vi "clusterUnderstanding.vi"() -> ()   [LabVIEW 2019]
panel:
  out "Numeric":dbl
  in  "Person  turn":dbl
  out "LED Two":bool
  out "Name":string
  out "Age":dbl
  out "LED One":bool
  in  "Cluster":T1
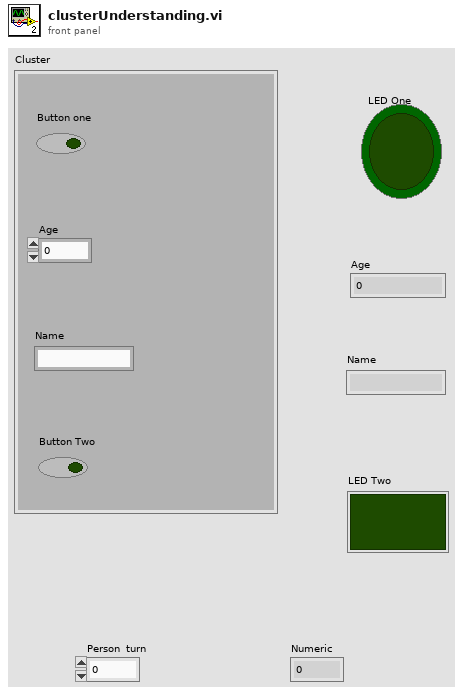
[diagram p1: front panel]
types:
  T1 = cluster{"Button one":bool, "Age":dbl, "Name":string, "Button Two ":bool}
  T2 = cluster{"Cluster":cluster{"Button one":bool, "Age":dbl, "Name":string, "Button Two ":bool}, "Person  turn":dbl}
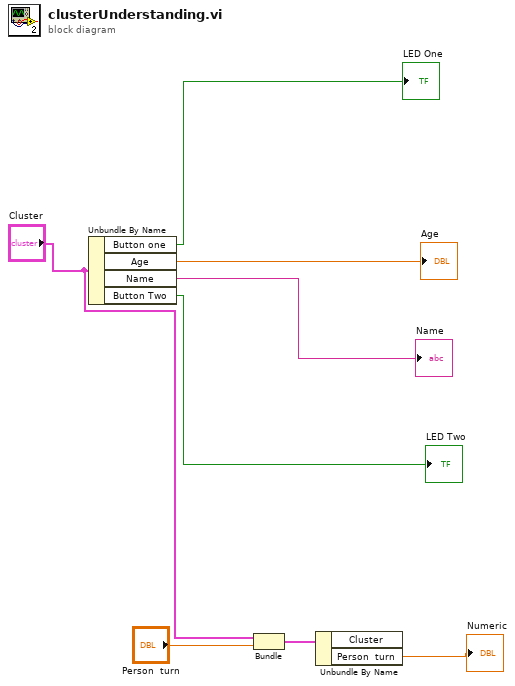
[diagram p0: block diagram]
diagram:
  n1 = Unbundle By Name("Cluster") -> ("Button one"=→"LED One":bool, "Age"=→"Age":dbl, "Name"=→"Name":string, "Button Two"=→"LED Two":bool)
  n2 = Bundle "Bundle"("Cluster"="Cluster", "Person  turn"="Person  turn") -> (w2:T2)  [unwired: 1 in]
  n3 = Unbundle By Name(w2) -> ("Person  turn"=→"Numeric":dbl)  [unwired: 1 out]
